vi "prepare_position_overlay.vi"(7 "progress bar ref":refnum<vi>, 8 "error in (no error)":errorcluster, 10 "position channels":T2, 11 "ImageCollection in":refnum<class "ImageCollection.lvclass">) -> (0 "error out":errorcluster, 2 "pixel positions":T1, 3 "ImageCollection out":refnum<class "ImageCollection.lvclass">)   [LabVIEW 2010, in "ImageCollection.lvclass"]
uses:
  ImageCollection.lvclass
  position_channels_cluster.ctl
  pixel_positions_cluster.ctl
  Image/Image/position_channels_cluster.ctl
  Image/Image/Image.lvclass
  ImageCollection.lvclass/ImageCollection.ctl
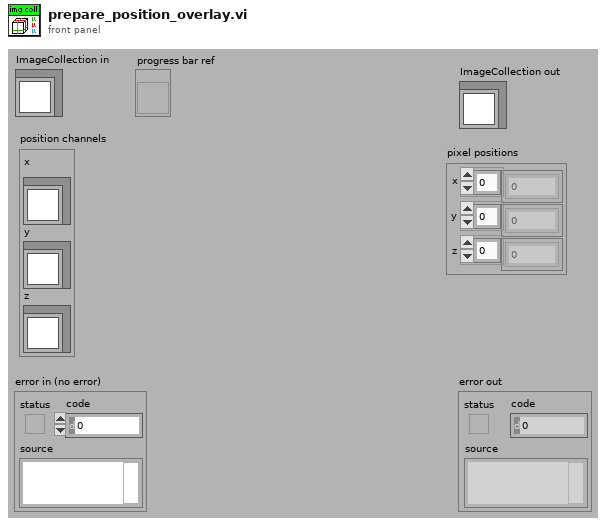
[diagram p1: front panel]
types:
  T1 = typedef "ImageCollection.lvclass/pixel_positions_cluster.ctl" = cluster{"x":dbl[], "y":dbl[], "z":dbl[]}
  T2 = typedef "ImageCollection.lvclass/position_channels_cluster.ctl" = cluster{"x":refnum<class "ImageCollection.lvclass">, "y":refnum<class "ImageCollection.lvclass">, "z":refnum<class "ImageCollection.lvclass">}
  T3 = typedef "Image.lvclass/position_channels_cluster.ctl" = cluster{"x":refnum<class "Image.lvclass">, "y":refnum<class "Image.lvclass">, "z":refnum<class "Image.lvclass">}
  T4 = typedef "Image Type" = u32
  T5 = cluster{"position channels[0]":refnum<class "ImageCollection.lvclass">, "position channels[1]":refnum<class "ImageCollection.lvclass">, "position channels[2]":refnum<class "ImageCollection.lvclass">}
  T6 = typedef "Image.lvclass/pixel_positions_cluster.ctl" = cluster{"x":dbl[], "y":dbl[], "z":dbl}
  T7 = cluster{"[0]":cluster{"mean values":dbl[]}, "[1]":cluster{"mean values":dbl[]}}
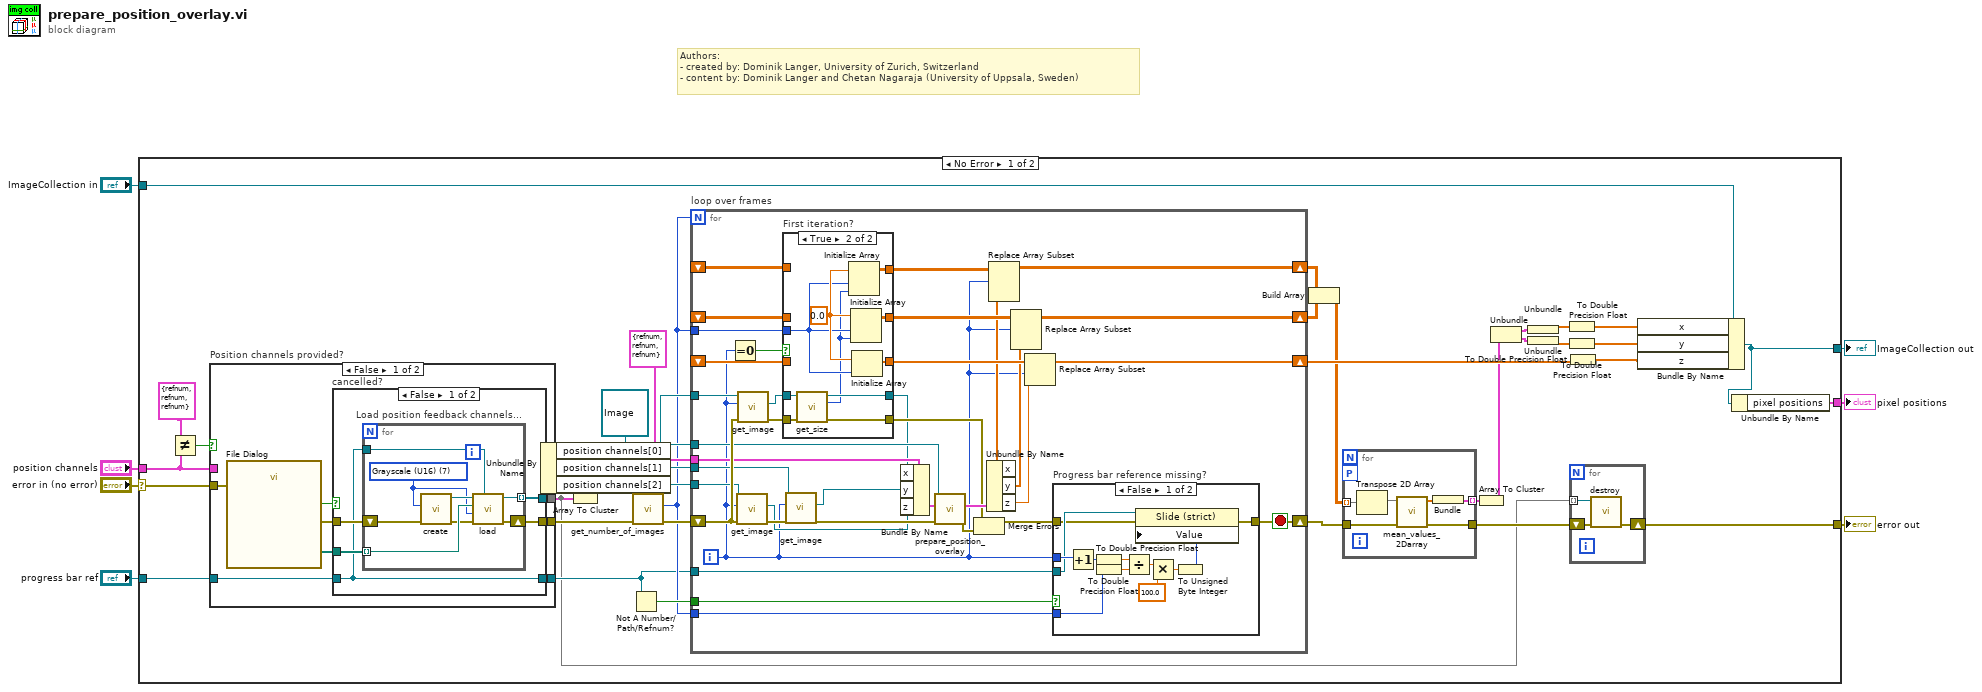
[diagram p0: block diagram]
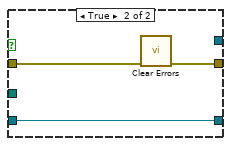
[diagram p2: hidden frame]
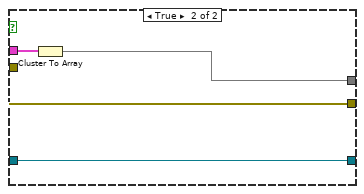
[diagram p3: hidden frame]
diagram:
  # "Authors: \n- created by: Dominik Langer, University of Zurich, Switzerland\n- content by: Dominik Langer and Chetan Nagaraja (University of Uppsala, Sweden)"
  n1 = case shown="No Error" "error in (no error)" {
    selector: "error in (no error)" -> [w14 w147]
    tunnel: [w10 w147] -> w6
    tunnel: [w18 w146] -> w4
    tunnel: "ImageCollection in" -> [w20 w146]
    tunnel: "position channels" -> [w13 _]
    tunnel: "progress bar ref" -> [w12 _]
    tunnel: [w26 _] -> w1
    frame No Error {
      n2 = Not Equal?(x=T2 {"x"=refnum, "y"=refnum, "z"=refnum} ("position channels"), y=w13) -> (x != y?=w16:bool)
      n3 = case "Position channels provided?" shown="False" w16 {
        tunnel: [w51 w74] -> w15
        tunnel: w14 -> [w50 w74]
        tunnel: [w49 w71] -> w8
        tunnel: w13 -> [_ w72]
        tunnel: w12 -> [w48 w73]
        tunnel: [w47 w73] -> _
        frame False {
          n4 = call "File Dialog"("error in"=w50) -> ("selected paths"=w53:path[], "cancelled"=w52:bool, "error out"=w54:errorcluster)  [unwired: 11 in, 1 out]
          n5 = case "cancelled?" shown="False" w52 {
            tunnel: w54 -> [w58 w70]
            tunnel: [w59 w69] -> w51
            tunnel: w53 -> [w57 _]
            tunnel: [w55 _] -> w49
            tunnel: w48 -> [w56 w68]
            tunnel: [w56 w68] -> w47
            frame False {
              n6 = for "Load position feedback channels..." {
                tunnel: [w67] -> w55 mode=indexing
                shift-right: [w66] -> w59
                shift-left: w58 -> [w65]
                tunnel: w57 -> [w64] mode=indexing
                tunnel: w56 -> [w63]
                w60 = T4 7 items=["Grayscale (U8)", "Grayscale (I16)", "Grayscale (SGL)", "Complex (CSG)", "RGB (U32)", "HSL (U32)", "RGB (U64)", "Grayscale (U16)"] ("Image Type")
                n7 = call "create.vi"("error in (no error)"=w65, "Image Type"=w60) -> ("error out"=w62:errorcluster, "ImageCollection out"=w61:refnum<class "ImageCollection.lvclass">)  [unwired: 8 in]
                n8 = call "load.vi"("progress bar ref"=w63, "error in (no error)"=w62, "Image Type"=w60, "path in"=w64, "ImageCollection in"=w61) -> ("error out"=w66:errorcluster, "ImageCollection out"=w67:refnum<class "ImageCollection.lvclass">)  [unwired: 2 in, 3 out]
              }
            }
            frame True {
              n9 = call <vilib>:"Clear Errors.vi"("error in (no error)"=w70) -> ("error out"=w69:errorcluster)  [unwired: 6 in]
            }
          }
        }
        frame True {
          n10 = Cluster To Array(cluster=w72) -> (array=w71:refnum<class "ImageCollection.lvclass">[])
        }
      }
      n11 = Array To Cluster(array=w8) -> (cluster=w11:T5)
      n12 = Unbundle By Name(w11) -> ("position channels[0]"=w37:refnum<class "ImageCollection.lvclass">, "position channels[1]"=w40:refnum<class "ImageCollection.lvclass">, "position channels[2]"=w39:refnum<class "ImageCollection.lvclass">)
      n13 = Not A Number/Path/Refnum?(number/path/refnum=w12) -> (NaN/Path/Refnum?=w23:bool)
      n14 = call-dynamic "get_number_of_images.vi"("error in (no error)"=w15, "ImageCollection in"=w37) -> ("error out"=w35:errorcluster, "size"=w22:i32, "ImageCollection out"=w36:refnum<class "ImageCollection.lvclass">)  [unwired: 7 in]
      n15 = for "loop over frames" {
        N: w22 -> [_]
        shift-right: [w116] -> w33
        shift-left: _ -> [w107]
        shift-right: [w117] -> w34
        shift-left: _ -> [w106]
        shift-right: [w115] -> w38
        shift-left: _ -> [w102]
        shift-right: [w81] -> w21
        shift-left: w35 -> [w114]
        tunnel: w36 -> [w113]
        tunnel: w40 -> [w112]
        tunnel: w39 -> [w111]
        tunnel: w22 -> [w109]
        tunnel: refnum<class "Image.lvclass"> refnum ("Image.lvclass") -> [w94]
        tunnel: T3 {"x"=refnum, "y"=refnum, "z"=refnum} ("position channels") -> [w91]
        tunnel: w12 -> [w83]
        tunnel: w23 -> [w82]
        tunnel: w22 -> [w84]
        i -> [w86]
        stop <- w81 stop-if-true
        n16 = Equal To 0?(x=w86) -> (x = 0?=w103:bool)
        n17 = call-dynamic "get_image.vi"("error in (no error)"=w114, "index"=w86, "ImageCollection in"=w111) -> ("error out"=w96:errorcluster, "Image.lvclass"=w89:refnum<class "Image.lvclass">)  [unwired: 6 in, 1 out]
        n18 = call-dynamic "get_image.vi"("error in (no error)"=w114, "index"=w86, "ImageCollection in"=w113) -> ("error out"=w105:errorcluster, "Image.lvclass"=w104:refnum<class "Image.lvclass">)  [unwired: 6 in, 1 out]
        n19 = case "First iteration?" shown="True" w103 {
          tunnel: w105 -> [w132 w145]
          tunnel: w104 -> [w133 w144]
          tunnel: [w135 w143] -> w110
          tunnel: w109 -> [_ w137]
          tunnel: [w134 w142] -> w108
          tunnel: w107 -> [w135 _]
          tunnel: w106 -> [w134 _]
          tunnel: [w132 w141] -> w93
          tunnel: [w133 w140] -> w87
          tunnel: w102 -> [w131 _]
          tunnel: [w131 w138] -> w101
          frame False {
          }
          frame True {
            w139 = 0.0 ("Numeric")
            n20 = call-dynamic "get_size.vi"("error in (no error)"=w145, "Image in"=w144) -> ("error out"=w141:errorcluster, "x resolution"=w136:i32, "Image out"=w140:refnum<class "Image.lvclass">)  [unwired: 2 in, 5 out]
            n21 = Initialize Array(w139, w137, w136) -> (w142:dbl[][])
            n22 = Initialize Array(w139, w137, w136) -> (w143:dbl[][])
            n23 = Initialize Array(w139, w137) -> (w138:dbl[])
          }
        }
        n24 = call-dynamic "get_image.vi"("error in (no error)"=w96, "index"=w86, "ImageCollection in"=w112) -> ("error out"=w95:errorcluster, "Image.lvclass"=w90:refnum<class "Image.lvclass">)  [unwired: 6 in, 1 out]
        n25 = Bundle By Name(cluster=w91, "x"=w87, "y"=w90, "z"=w89) -> (w88:T3)
        n26 = call "prepare_position_overlay.vi"("error in (no error)"=w95, "position channels"=w88, "Image in"=w94) -> ("error out"=w92:errorcluster, "pixel positions"=w100:T6)  [unwired: 6 in, 1 out]
        n27 = Merge Errors(w93, w92) -> (w85:errorcluster)
        n28 = Unbundle By Name(w100) -> ("x"=w99:dbl[], "y"=w98:dbl[], "z"=w97:dbl)
        n29 = Replace Array Subset(array=w108, new element=w99, index (row)=w86) -> (w117:dbl[][])  [unwired: 1 in]
        n30 = Replace Array Subset(array=w110, new element=w98, index (row)=w86) -> (w116:dbl[][])  [unwired: 1 in]
        n31 = Replace Array Subset(array=w101, new element=w97, index=w86) -> (w115:dbl[])
        n32 = case "Progress bar reference missing?" shown="False" w82 {
          tunnel: w84 -> [w125 _]
          tunnel: w86 -> [w122 _]
          tunnel: w83 -> [w121 _]
          tunnel: w85 -> [w120 w130]
          tunnel: [w119 w130] -> w81
          frame False {
            n33 = Increment(x=w122) -> (x+1=w123:i32)
            n34 = To Double Precision Float(number=w123) -> (double precision float=w126:dbl)
            n35 = To Double Precision Float(number=w125) -> (double precision float=w124:dbl)
            n36 = Divide(x=w126, y=w124) -> (x/y=w129:dbl)
            n37 = Multiply(x=w129, y=100.0) -> (x*y=w127:dbl)
            n38 = To Unsigned Byte Integer(number=w127) -> (unsigned 8bit integer=w118:u8)
            n39 = property class="Slide (strict)"(reference=w121, error in=w120, "Value"=w118) -> (error out=w119:errorcluster)  [unwired: 1 out]
          }
          frame True {
          }
        }
      }
      n40 = Build Array(w34, w33) -> (w32:dbl[][][])
      n41 = for {
        tunnel: [w76] -> w31 mode=indexing
        tunnel: w32 -> [w80] mode=indexing
        workers-P: _ -> [_]
        tunnel: w21 -> [w78]
        tunnel: [w75] -> w9
        n42 = Transpose 2D Array(2D array=w80) -> (transposed array=w79:dbl[][])
        n43 = call "mean_values_2Darray.vi"("error in (no error)"=w78, "Array"=w79) -> ("error out"=w75:errorcluster, "mean values"=w77:dbl[])  [unwired: 6 in]
        n44 = Bundle("mean values"=w77) -> (w76:cluster{"mean values":dbl[]})  [unwired: 1 in]
      }
      n45 = Array To Cluster(array=w31) -> (cluster=w19:T7)
      n46 = Unbundle(w19) -> ("[0]"=w30:cluster{"mean values":dbl[]}, "[1]"=w28:cluster{"mean values":dbl[]})
      n47 = Unbundle(w30) -> ("mean values"=w29:dbl[])
      n48 = Unbundle(w28) -> ("mean values"=w27:dbl[])
      n49 = To Double Precision Float(number=w29) -> (double precision float=w43:dbl[])
      n50 = To Double Precision Float(number=w27) -> (double precision float=w42:dbl[])
      n51 = To Double Precision Float(number=w38) -> (double precision float=w41:dbl[])
      n52 = for {
        shift-right: [w46] -> w10
        shift-left: w9 -> [w45]
        tunnel: w8 -> [w44] mode=indexing
        n53 = call-dynamic "destroy.vi"("error in (no error)"=w45, "ImageCollection in"=w44) -> ("error out"=w46:errorcluster)  [unwired: 8 in, 1 out]
      }
      n54 = Bundle By Name(cluster=w20, "x"=w43, "y"=w42, "z"=w41) -> (w18:refnum<class "ImageCollection.lvclass">)
      n55 = Unbundle By Name(w18) -> ("pixel positions"=w26:T1)
    }
    frame Error {
    }
  }
  "error out" <- w6
  "ImageCollection out" <- w4
  "pixel positions" <- w1
